vi "Data Access.vi"(8 "error in (no error)":errorcluster, 10 "Data Access Handler":refnum<class "Data Access Handler.lvclass">, 11 "DMM Config RTD Type Msg in":refnum<class "DMM Config RTD Type Msg.lvclass">) -> (0 "error out":errorcluster, 3 "DMM Config RTD Type out":refnum<class "DMM Config RTD Type Msg.lvclass">)   [LabVIEW 2020, in "DMM Msg.lvlib" / "DMM Config RTD Type Msg.lvclass"]
doc: "Expose class private data to the front panel while letting the Data Access Handler class act on the data."
uses:
  DMM Config RTD Type Msg.lvclass
  C:/Current projects/WS/PPL/HDH.Actor Framework.Core.Msg.lvlibp/Flex Msg/Flex Msg.lvclass
  PPL/HDH.Actor Framework.Core.Msg.lvlibp/Flex Msg/Data Access Handlers/Data Access Handler/Data Access Handler.lvclass
  PPL/HDH.Actor Framework.Core.Publisher.lvlibp/Messages/Response Msg/Response Core/Controls/Ctl_SendFunction.ctl
  PPL/HDH.Driver.DMM.lvlibp/Controls/Ctl_RTDType.ctl
  DMM Config RTD Type Msg.lvclass/DMM Config RTD Type Msg.ctl
  PPL/HDH.Actor Framework.Core.Instrument Handler.lvlibp/Messages/Instrument Msg/Instrument Msg.lvclass
  C:/Current projects/WS/PPL/HDH.Actor Framework.Core.Instrument Handler.lvlibp/Messages/Instrument Msg/Instrument Msg.lvclass
  PPL/HDH.Driver.DMM.lvlibp
  PPL/HDH.Actor Framework.Core.Publisher.lvlibp
panel:
  in  "Resistance at 0°C":dbl=100.0
  in  "RTD Type":T1=enum."Pt3851"
  in  "Message Priority":enum16{"Low", "Normal", "High"}(ring)=enum."Normal"
  in  "Timeout if Waiting":i32=-1
  in  "Send Function":T2=enum."Await Reply"
  in  "Cancel":bool
  in  "OK":bool
  # "Send details"
  # "RTD Type Configuration details"
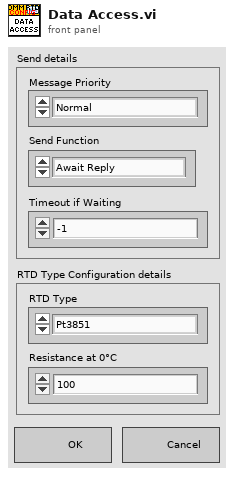
[diagram p1: front panel]
types:
  T1 = typedef "HDH.Driver.DMM.lvlibp/Ctl_RTDType.ctl" = enum16{"Custom", "Pt3750", "Pt3851", "Pt3911", "Pt3916", "Pt3920", "Pt3928"}
  T2 = typedef "HDH.Actor Framework.Core.Publisher.lvlibp/Ctl_SendFunction.ctl" = enum16{"Send and Forget", "Request Reply", "Await Reply"}
  T3 = typedef "HDH.Actor Framework.Core.Actor.lvlibp/Message Enqueuer.lvclass/Message Priority.ctl" = enum16{"Low", "Normal", "High"}
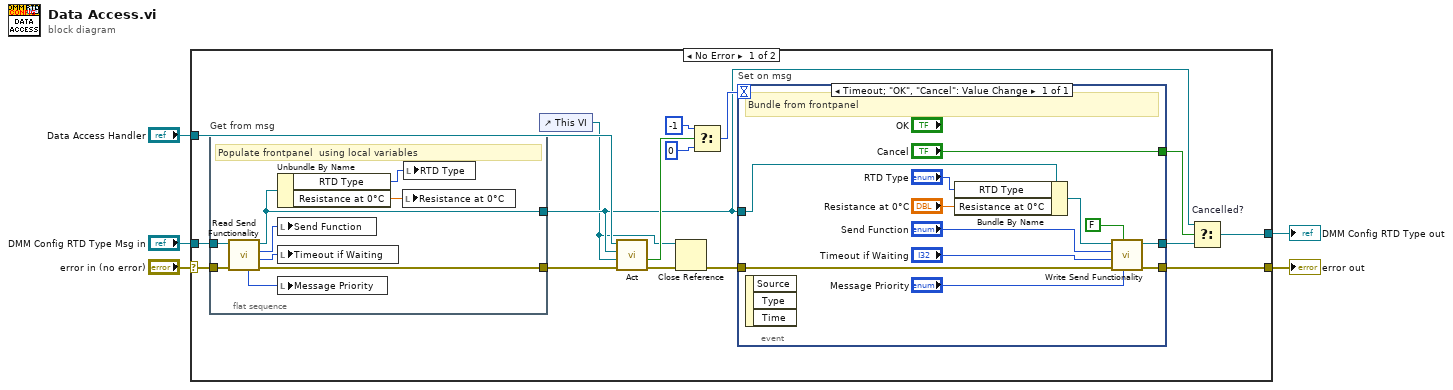
[diagram p0: block diagram]
diagram:
  n1 = case shown="No Error" "error in (no error)" {
    selector: "error in (no error)" -> [w21 w44]
    tunnel: [w14 w44] -> w4
    tunnel: [w9 w43] -> w2
    tunnel: "DMM Config RTD Type Msg in" -> [w12 w43]
    tunnel: "Data Access Handler" -> [w20 _]
    frame No Error {
      n2 = flat-sequence "Get from msg" {
        tunnel: w21 -> [w41]
        tunnel: [w39] -> w7
        tunnel: w12 -> [w42]
        tunnel: [w40] -> w19
        frame #0 {
          # "Populate frontpanel  using local variables"
          n3 = call "Read Send Functionality.vi"("error in (no error)"=w41, "Instrument Msg in"=w42) -> ("error out"=w40:errorcluster, "Timeout if Waiting"=w37:i32, "Send Function"=w38:T2, "Instrument Msg out"=w39:refnum<class "DMM Config RTD Type Msg.lvclass">, "Message Priority"=w36:T3)  [unwired: 4 in, 1 out]
          n4 = Unbundle By Name(w39) -> ("RTD Type"=w35:T1, "Resistance at 0°C"=w34:dbl)
          n5 = local write "Send Function"(w38) -> ()
          n6 = local write "Timeout if Waiting"(w37) -> ()
          n7 = local write "Message Priority"(w36) -> ()
          n8 = local write "Resistance at 0°C"(w34) -> ()
          n9 = local write "RTD Type"(w35) -> ()
        }
      }
      n10 = control-ref of="This VI"() -> (w6:refnum<vi>)
      n11 = call-dynamic "Act.vi"("error in (no error)"=w19, "VI Refnum in"=w6, "Flex Msg type"=w7, "Data Access Handler in"=w20) -> ("error out"=w11:errorcluster, "Await user action?"=w18:bool)  [unwired: 5 in, 1 out]
      n12 = Close Reference(reference=w6, error in (no error)=w11) -> (error out=w13:errorcluster)
      n13 = Select(t=-1, s=w18, f=0 ("t")) -> (s? t:f=w15:i32)
      n14 = event "Set on msg" shown="[0] Timeout;  \"OK\", \"Cancel\": Value Change" {
        selector: _ -> [_]
        dyn-events: _ -> [_]
        timeout: w15 -> [_]
        tunnel: [w28] -> w14
        tunnel: w13 -> [w29]
        tunnel: ["Cancel"] -> w10
        tunnel: [w31] -> w8
        tunnel: w7 -> [w32]
        event Timeout; "OK", "Cancel": Value Change {
          # "Bundle from frontpanel"
          n15 = event-data() -> ()  [unwired: 1 in, 3 out]
          n16 = Bundle By Name(cluster=w32, "RTD Type"="RTD Type", "Resistance at 0°C"="Resistance at 0°C") -> (w30:refnum<class "DMM Config RTD Type Msg.lvclass">)
          n17 = call "Write Send Functionality.vi"("Message Priority(Normal)"="Message Priority", "Publish Data?(T)"=FALSE, "error in (no error)"=w29, "Timeout if Waiting(-1ms)"="Timeout if Waiting", "Send Function(Await Reply)"="Send Function", "Instrument Msg in"=w30) -> ("error out"=w28:errorcluster, "Instrument Msg out"=w31:refnum<class "DMM Config RTD Type Msg.lvclass">)  [unwired: 4 in]
        }
      }
      n18 = Select "Cancelled?"(t=w7, s=w10, f=w8) -> (s? t:f=w9:refnum<class "DMM Config RTD Type Msg.lvclass">)
    }
    frame Error {
    }
  }
  "error out" <- w4
  "DMM Config RTD Type out" <- w2
